vi "Launcher.vi"() -> ()   [LabVIEW 2024]
doc: "UI API Tester."
uses:
  <vilib>/Utility/error.llb/DialogType.ctl
  Vending Machine/Libraries/UI/UI.lvlib
  Vending Machine/Libraries/Launcher Support/Launcher Support.lvlib
panel:
  in  "UI API TESTER":bool
  in  "Message API TESTER":bool
  in  "Product Contro API TESTER":bool
  in  "Money Contro API TESTER":bool
  out "last error":errorcluster
  in  "Show Diagram on Init":bool
  in  "Stop Module":bool
  in  "Start Module":bool
  out "Status":string
  out "Module Running?":bool
  # "This VI tests the API for the Module."
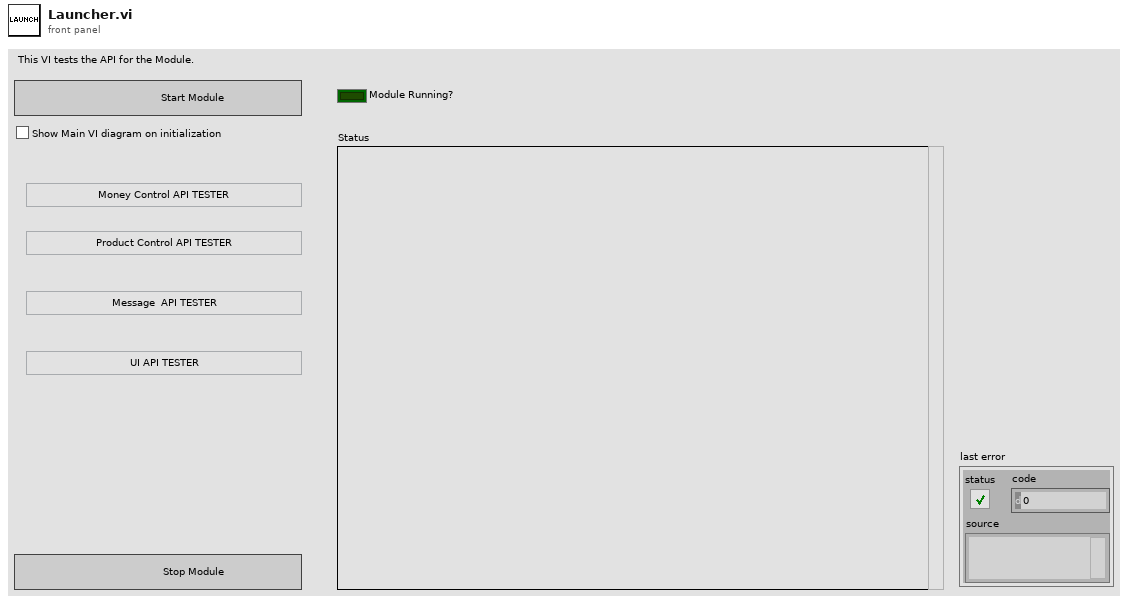
[diagram p1: front panel]
types:
  T1 = typedef "UI.lvlib/Broadcast Events--cluster.ctl" = cluster{"Module Did Init":refnum<user-event>, "Status Updated":refnum<user-event>, "Error Reported":refnum<user-event>, "Module Did Stop":refnum<user-event>, "Update Module Execution Status":refnum<user-event>}
  T2 = enum32{"invalid app kind", "Development System", "Run Time System", "Student Edition", "Embedded LabVIEW", "Evaluation", "Custom"}
  T3 = typedef "DialogType.ctl" = u16
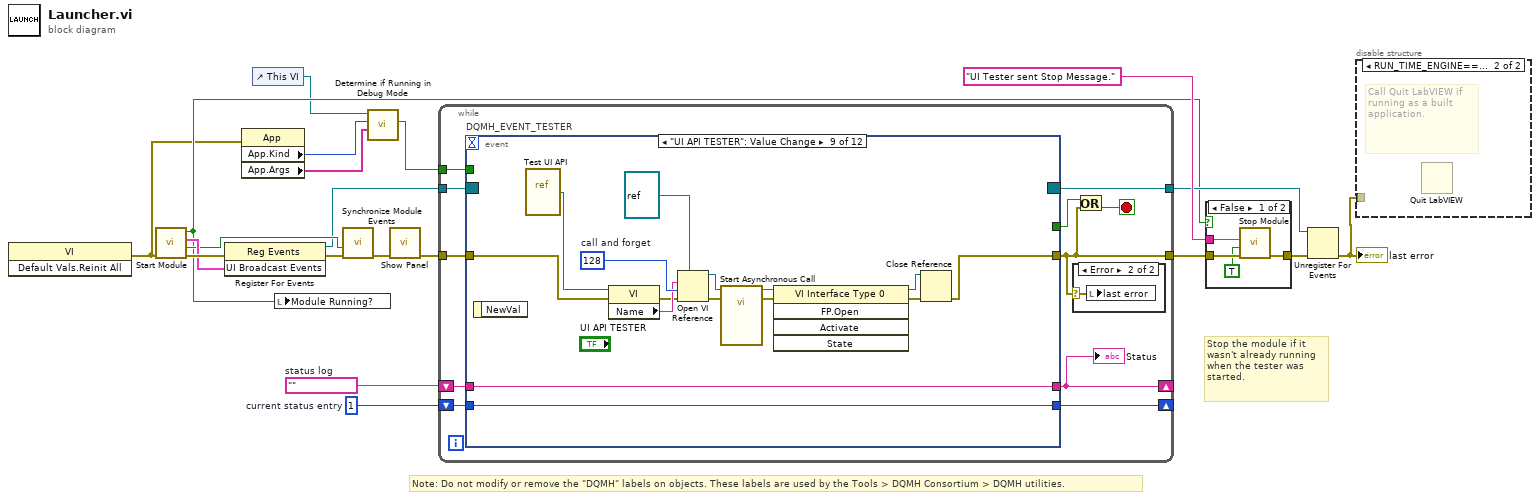
[diagram p0: block diagram]
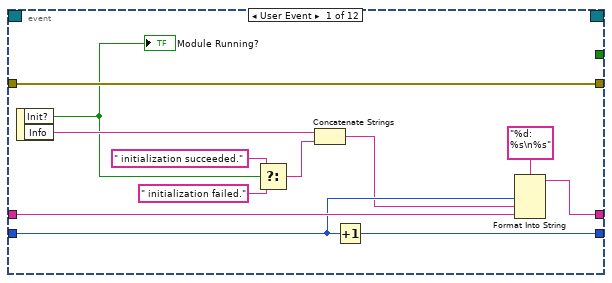
[diagram p5: hidden frame]
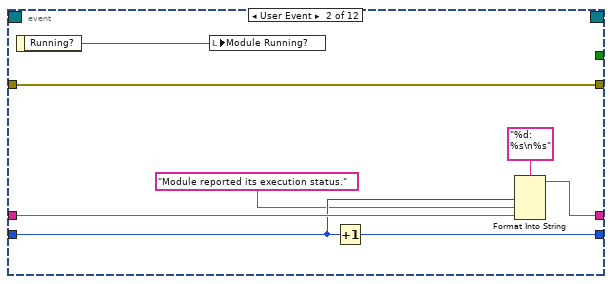
[diagram p6: hidden frame]
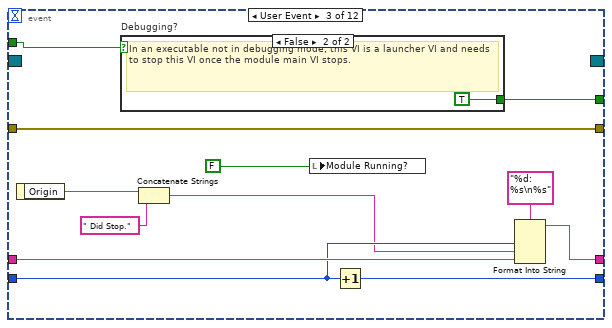
[diagram p7: hidden frame]
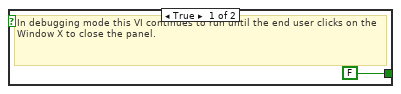
[diagram p8: hidden frame]
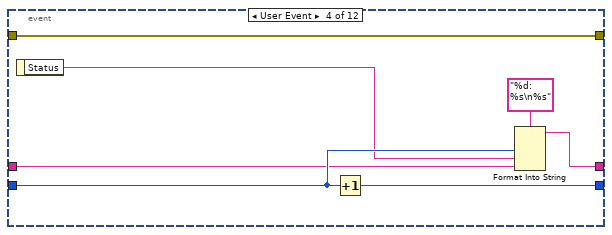
[diagram p9: hidden frame]
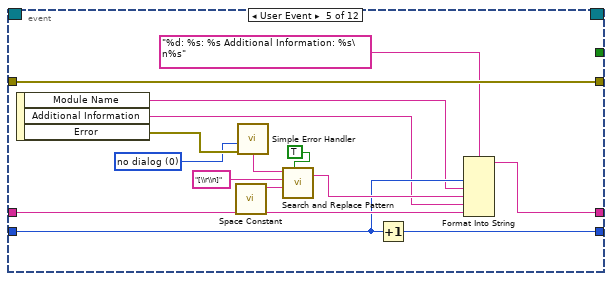
[diagram p10: hidden frame]
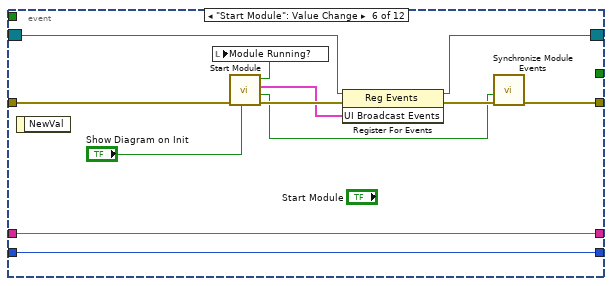
[diagram p11: hidden frame]
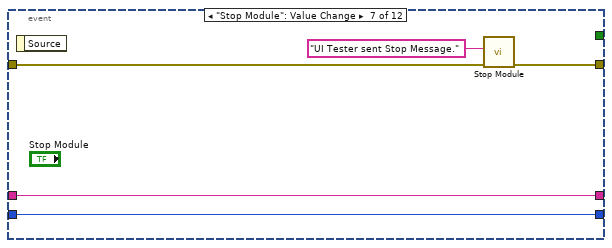
[diagram p12: hidden frame]
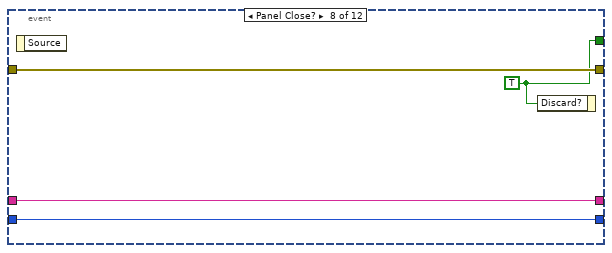
[diagram p13: hidden frame]
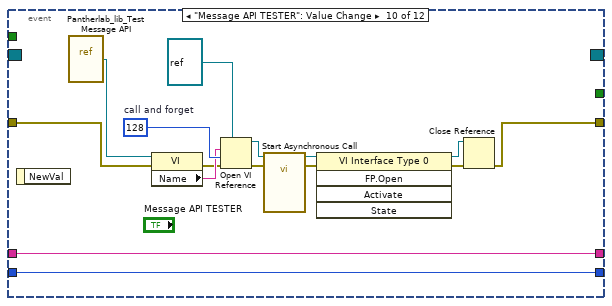
[diagram p14: hidden frame]
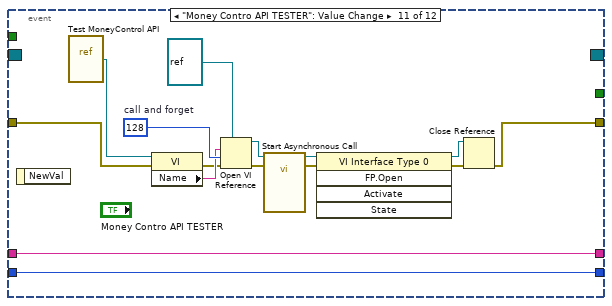
[diagram p15: hidden frame]
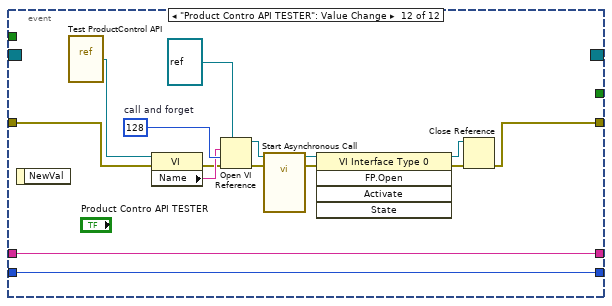
[diagram p16: hidden frame]
diagram:
  w12 = 1  # current status entry
  w13 = ""  # status log
  # "Stop the module if it wasn't already running when the tester was started."
  # "Note: Do not modify or remove the \"DQMH\" labels on objects. These labels are used by the Tools > DQMH Consortium > DQMH utilities."
  n1 = invoke class="VI" method="Default Vals.Reinit All"() -> (error out=w5:errorcluster)  [unwired: 3 in, 2 out]
  n2 = call "Start Module.vi"("error in"=w5) -> ("error out"=w17:errorcluster, "Wait for Event Sync?"=w9:bool, "UI Broadcast Events"=w10:T1, "Module Was Already Running?"=w7:bool)  [unwired: 6 in, 1 out]
  n3 = register-events(error in=w17, w10) -> (reference out=w8:refnum<event-registration>, error out=w18:errorcluster)  [unwired: 1 in]
  n4 = property on="Property Node" class="App"(error in=w5) -> ("App.Kind"=w4:T2, "App.Args"=w3:string[])  [unwired: 1 in, 2 out]
  n5 = control-ref of="This VI"() -> (w6:refnum<vi>)
  n6 = local write "Module Running?"(w7) -> ()
  n7 = call "Synchronize Module Events.vi"("error in"=w18, "Wait for Event Sync?"=w9) -> ("error out"=w16:errorcluster)  [unwired: 9 in]
  n8 = call "Determine if Running in Debug Mode.vi"("App.Args"=w3, "App.Kind"=w4, "Launcher VI ref"=w6) -> ("Debug mode?"=w2:bool)  [unwired: 8 in]
  n9 = call "Show Panel.vi"("error in"=w16) -> ("error out"=w15:errorcluster)  [unwired: 10 in]
  n10 = while {
    tunnel: [w21] -> w19
    shift-right: [w27] -> _
    shift-left: w13 -> [w29]
    shift-right: [w28] -> _
    shift-left: w12 -> [w30]
    tunnel: [w26] -> w11
    tunnel: w15 -> [w31]
    tunnel: w8 -> [w25]
    tunnel: w2 -> [w24]
    stop <- w23 stop-if-true
    n11 = event "DQMH_EVENT_TESTER" shown="[8] \"UI API TESTER\": Value Change" {
      selector: w25 -> [_ _ _ _ _ w92 _ _ _ _ _ _]
      dyn-events: [_ _ _ _ _ w91 _ _ _ _ _ _] -> w26
      timeout: _ -> [_ _ _ _ _ _ _ _ _ _ _ _]
      tunnel: [w44 w52 w64 w73 w87 w98 w105 w109 w112 w127 w142 w157] -> w21
      tunnel: w30 -> [w41 w49 w61 w69 w78 w95 w103 w107 w123 w138 w153 w168]
      tunnel: w29 -> [w42 w50 w62 w68 w79 w96 w104 w108 w124 w139 w154 w169]
      tunnel: [w39 w47 w59 w70 w77 w96 w104 w108 w124 w139 w154 w169] -> w27
      tunnel: [w40 w48 w60 w72 w76 w95 w103 w107 w123 w138 w153 w168] -> w28
      tunnel: w31 -> [w44 w52 w64 w73 w87 w97 w101 w109 w111 w126 w141 w156]
      tunnel: w24 -> [_ _ w54 _ _ _ _ _ _ _ _ _]
      tunnel: [_ _ w53 _ _ _ _ w106 _ _ _ _] -> w22
      event User Event {
        n12 = event-data() -> ("Init?"=w36:bool, "Info"=w38:string)  [unwired: 1 in]
        "Module Running?" <- w36
        n13 = Select(t=" initialization succeeded.", s=w36, f=" initialization failed.") -> (s? t:f=w33:string)
        n14 = Concatenate Strings(w38, w33) -> (w37:string)
        n15 = Increment(x=w41) -> (x+1=w40:i32)
        n16 = Format Into String(format string="%d: %s\n%s", w41, w37, w42) -> (resulting string=w39:string)  [unwired: 2 in, 1 out]
      }
      event User Event {
        n17 = event-data() -> ("Running?"=w45:bool)  [unwired: 1 in]
        n18 = local write "Module Running?"(w45) -> ()
        n19 = Increment(x=w49) -> (x+1=w48:i32)
        n20 = Format Into String(format string="%d: %s\n%s", w49, "Module reported its execution status.", w50) -> (resulting string=w47:string)  [unwired: 2 in, 1 out]
      }
      event User Event {
        n21 = event-data() -> ("Origin"=w58:string)  [unwired: 1 in]
        n22 = case "Debugging?" shown="False" w54 {
          tunnel: [FALSE ("Discard?") TRUE ("Discard?")] -> w53
          frame True {
            # "In debugging mode this VI continues to run until the end user clicks on the Window X to close the panel."
          }
          frame False {
            # "In an executable not in debugging mode, this VI is a launcher VI and needs to stop this VI once the module main VI stops."
          }
        }
        n23 = Concatenate Strings(w58, " Did Stop.") -> (w57:string)
        n24 = local write "Module Running?"(FALSE ("Module Did Init?")) -> ()
        n25 = Increment(x=w61) -> (x+1=w60:i32)
        n26 = Format Into String(format string="%d: %s\n%s", w61, w57, w62) -> (resulting string=w59:string)  [unwired: 2 in, 1 out]
      }
      event User Event {
        n27 = event-data() -> ("Status"=w67:string)  [unwired: 1 in]
        n28 = Increment(x=w69) -> (x+1=w72:i32)
        n29 = Format Into String(format string="%d: %s\n%s", w69, w67, w68) -> (resulting string=w70:string)  [unwired: 2 in, 1 out]
      }
      event User Event {
        w80 = T3 0 items=["no dialog", "OK message", "continue or stop message", "OK message + warnings", "continue/stop + warnings"] ("type of dialog (OK msg:1)")
        n30 = event-data() -> ("Module Name"=w75:string, "Additional Information"=w74:string, "Error"=w88:errorcluster)  [unwired: 1 in]
        n31 = call <vilib>:"Space Constant.vi"() -> ("String"=w84:string)
        n32 = call <vilib>:"Simple Error Handler.vi"("type of dialog (OK msg:1)"=w80, "error in (no error)"=w88) -> ("message"=w81:string)  [unwired: 3 in, 4 out]
        n33 = call <vilib>:"Search and Replace Pattern.vi"("string"=w81, "regular expression (\"\")"="[\\r\\n]" ("regular expression (\"\")"), "replace string (\"\")"=w84, "replace all? (F)"=TRUE ("replace all CR/LF with spaces")) -> ("result string"=w82:string)  [unwired: 1 in, 1 out]
        n34 = Increment(x=w78) -> (x+1=w76:i32)
        n35 = Format Into String(format string="%d: %s: %s Additional Information: %s\n%s", w78, w75, w82, w74, w79) -> (resulting string=w77:string)  [unwired: 2 in, 1 out]
      }
      event "Start Module": Value Change {
        n36 = event-data() -> ()  [unwired: 1 in, 1 out]
        n37 = call "Start Module.vi"("Show Main VI Diagram on Init (F)"="Show Diagram on Init", "error in"=w97) -> ("error out"=w99:errorcluster, "Wait for Event Sync?"=w94:bool, "UI Broadcast Events"=w93:T1, "Module Was Already Running?"=w90:bool)  [unwired: 5 in, 1 out]
        n38 = local write "Module Running?"(w90) -> ()
        n39 = register-events(reference=w92, error in=w99, w93) -> (reference out=w91:refnum<event-registration>, error out=w100:errorcluster)
        n40 = call "Synchronize Module Events.vi"("error in"=w100, "Wait for Event Sync?"=w94) -> ("error out"=w98:errorcluster)  [unwired: 9 in]
      }
      event "Stop Module": Value Change {
        n41 = event-data() -> ()  [unwired: 1 in, 1 out]
        n42 = call "Stop Module.vi"("error in"=w101, "Origin"="UI Tester sent Stop Message.") -> ("error out"=w105:errorcluster)  [unwired: 9 in]
      }
      event Panel Close? {
        w106 = TRUE ("Discard?")
        n43 = event-data() -> ()  [unwired: 1 in, 1 out]
        n44 = event-data("Discard?"=w106) -> ()  [unwired: 1 in, 1 out]
      }
      event "UI API TESTER": Value Change {
        w122 = 128  # call and forget
        n45 = event-data() -> ()  [unwired: 1 in, 1 out]
        n46 = vi-ref "Test UI API.vi"() -> (w110:refnum<vi>)
        n47 = property class="VI"(reference=w110, error in=w111) -> (error out=w113:errorcluster, "Name"=w115:string)  [unwired: 1 out]
        n48 = Open VI Reference(type specifier VI Refnum (for type only)=refnum<vi> refnum, vi path=w115, options=w122, error in (no error)=w113) -> (vi reference=w118:refnum<vi>, error out=w114:errorcluster)  [unwired: 2 in]
        n49 = call-by-ref "Start Asynchronous Call"(reference=w118, error in=w114) -> (reference out=w120:refnum<vi>, error out=w117:errorcluster)  [unwired: 12 in]
        n50 = invoke class="VI Interface Type 0" method="FP.Open"(reference=w120, error in=w117) -> (reference out=w121:refnum<vi>, error out=w119:errorcluster)  [unwired: 3 in, 3 out]
        n51 = Close Reference(reference=w121, error in (no error)=w119) -> (error out=w112:errorcluster)
      }
      event "Message API TESTER": Value Change {
        w137 = 128  # call and forget
        n52 = event-data() -> ()  [unwired: 1 in, 1 out]
        n53 = vi-ref <vilib>:"Pantherlab_lib_Test Message API.vi"() -> (w125:refnum<vi>)
        n54 = property class="VI"(reference=w125, error in=w126) -> (error out=w128:errorcluster, "Name"=w130:string)  [unwired: 1 out]
        n55 = Open VI Reference(type specifier VI Refnum (for type only)=refnum<vi> refnum, vi path=w130, options=w137, error in (no error)=w128) -> (vi reference=w133:refnum<vi>, error out=w129:errorcluster)  [unwired: 2 in]
        n56 = call-by-ref "Start Asynchronous Call"(reference=w133, error in=w129) -> (reference out=w135:refnum<vi>, error out=w132:errorcluster)  [unwired: 12 in]
        n57 = invoke class="VI Interface Type 0" method="FP.Open"(reference=w135, error in=w132) -> (reference out=w136:refnum<vi>, error out=w134:errorcluster)  [unwired: 3 in, 3 out]
        n58 = Close Reference(reference=w136, error in (no error)=w134) -> (error out=w127:errorcluster)
      }
      event "Money Contro API TESTER": Value Change {
        w152 = 128  # call and forget
        n59 = event-data() -> ()  [unwired: 1 in, 1 out]
        n60 = vi-ref "Test MoneyControl API.vi"() -> (w140:refnum<vi>)
        n61 = property class="VI"(reference=w140, error in=w141) -> (error out=w143:errorcluster, "Name"=w145:string)  [unwired: 1 out]
        n62 = Open VI Reference(type specifier VI Refnum (for type only)=refnum<vi> refnum, vi path=w145, options=w152, error in (no error)=w143) -> (vi reference=w148:refnum<vi>, error out=w144:errorcluster)  [unwired: 2 in]
        n63 = call-by-ref "Start Asynchronous Call"(reference=w148, error in=w144) -> (reference out=w150:refnum<vi>, error out=w147:errorcluster)  [unwired: 12 in]
        n64 = invoke class="VI Interface Type 0" method="FP.Open"(reference=w150, error in=w147) -> (reference out=w151:refnum<vi>, error out=w149:errorcluster)  [unwired: 3 in, 3 out]
        n65 = Close Reference(reference=w151, error in (no error)=w149) -> (error out=w142:errorcluster)
      }
      event "Product Contro API TESTER": Value Change {
        w167 = 128  # call and forget
        n66 = event-data() -> ()  [unwired: 1 in, 1 out]
        n67 = vi-ref "Test ProductControl API.vi"() -> (w155:refnum<vi>)
        n68 = property class="VI"(reference=w155, error in=w156) -> (error out=w158:errorcluster, "Name"=w160:string)  [unwired: 1 out]
        n69 = Open VI Reference(type specifier VI Refnum (for type only)=refnum<vi> refnum, vi path=w160, options=w167, error in (no error)=w158) -> (vi reference=w163:refnum<vi>, error out=w159:errorcluster)  [unwired: 2 in]
        n70 = call-by-ref "Start Asynchronous Call"(reference=w163, error in=w159) -> (reference out=w165:refnum<vi>, error out=w162:errorcluster)  [unwired: 12 in]
        n71 = invoke class="VI Interface Type 0" method="FP.Open"(reference=w165, error in=w162) -> (reference out=w166:refnum<vi>, error out=w164:errorcluster)  [unwired: 3 in, 3 out]
        n72 = Close Reference(reference=w166, error in (no error)=w164) -> (error out=w157:errorcluster)
      }
    }
    "Status" <- w27
    n73 = case shown="Error" w21 {
      selector: w21 -> [_ w32]
      frame No Error {
      }
      frame Error {
        n74 = local write "last error"(w32) -> ()
      }
    }
    n75 = Or(x=w22, y=w21) -> (x .or. y?=w23:bool)
  }
  n76 = case shown="False" w7 {
    tunnel: [w173 w174] -> w20
    tunnel: "UI Tester sent Stop Message." ("Origin") -> [w171 _]
    tunnel: w19 -> [w172 w174]
    frame False {
      n77 = call "Stop Module.vi"("error in"=w172, "Wait for Module to Stop? (F)"=TRUE ("Wait for Module to stop?"), "Origin"=w171) -> ("error out"=w173:errorcluster)  [unwired: 8 in]
    }
    frame True {
    }
  }
  n78 = Unregister For Events(event registration refnum=w11, error in=w20) -> (error out=w1:errorcluster)
  "last error" <- w1
  n79 = disable-structure "Conditional Disable Structure" shown="RUN_TIME_ENGINE==True" {
    disable-tunnel: w1 -> [_ _]
    frame condition #0 (active) {
    }
    frame condition #1 {
      # "Call Quit LabVIEW if running as a built application."
      n80 = Quit LabVIEW() -> ()  [unwired: 1 in]
    }
  }
